vi "Initialize.vi"(7 "laserSettings":T1, 8 "error in (no error)":errorcluster, 10 "dllPath":path, 11 "serialNumber":string) -> (0 "error out":errorcluster, 3 "Laser Diode Controller out":refnum<class "KLD101.lvclass">)   [LabVIEW 2016, in "Laser Diode Controller.lvlib" / "KLD101.lvclass"]
uses:
  KLD101.lvclass
  TypeDefs/KLD-LaserSettings.ctl
  TypeDefs/KLD-LaserMode.ctl
  TypeDefs/KLD-LaserPolarity.ctl
  TypeDefs/KLD-LaserRampMode.ctl
  KLD101.lvclass/KLD101.ctl
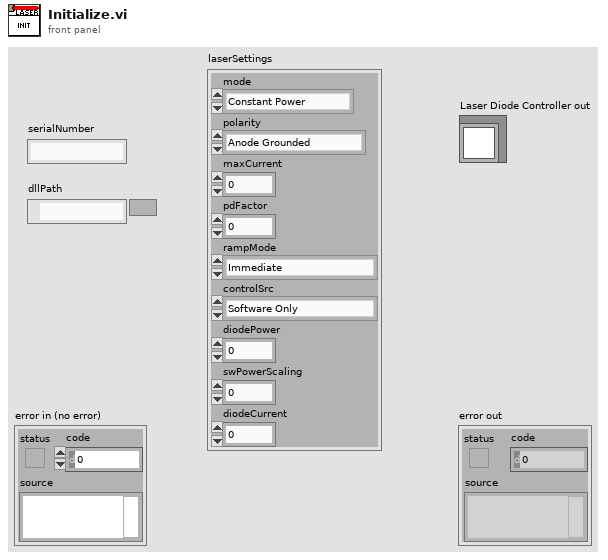
[diagram p1: front panel]
types:
  T1 = typedef "Laser Diode Controller.lvlib/KLD101.lvclass/KLD-LaserSettings.ctl" = cluster{"mode":T2, "polarity":T3, "maxCurrent":i16, "pdFactor":sgl, "rampMode":T4, "controlSrc":enum16{"Software Only", "External Signal", "Potentiometer"}, "diodePower":dbl, "swPowerScaling":dbl, "diodeCurrent":dbl}
  T2 = typedef "Laser Diode Controller.lvlib/KLD101.lvclass/KLD-LaserMode.ctl" = enum16{"Constant Power", "Constant Current"}
  T3 = typedef "Laser Diode Controller.lvlib/KLD101.lvclass/KLD-LaserPolarity.ctl" = enum16{"Anode Grounded", "Cathode Grounded"}
  T4 = typedef "Laser Diode Controller.lvlib/KLD101.lvclass/KLD-LaserRampMode.ctl" = enum16{"Immediate", "Ramped"}
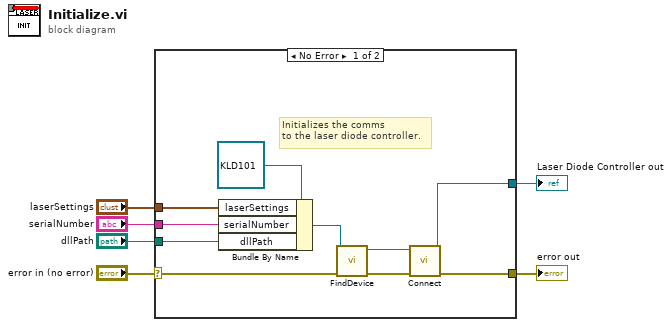
[diagram p0: block diagram]
diagram:
  n1 = case shown="No Error" "error in (no error)" {
    selector: "error in (no error)" -> [w12 w17]
    tunnel: [w8 w17] -> w5
    tunnel: [w10 _] -> w4
    tunnel: "serialNumber" -> [w13 _]
    tunnel: "laserSettings" -> [w15 _]
    tunnel: "dllPath" -> [w7 _]
    frame No Error {
      # "Initializes the comms\nto the laser diode controller."
      n2 = Bundle By Name(cluster=refnum<class "KLD101.lvclass"> refnum ("Laser Diode Controller out"), "laserSettings"=w15, "serialNumber"=w13, "dllPath"=w7) -> (w14:refnum<class "KLD101.lvclass">)
      n3 = call-dynamic "FindDevice.vi"("error in (no error)"=w12, "Laser Diode Controller in"=w14) -> ("error out"=w9:errorcluster, "Laser Diode Controller out"=w11:refnum<class "KLD101.lvclass">)  [unwired: 8 in]
      n4 = call-dynamic "Connect.vi"("error in (no error)"=w9, "Laser Diode Controller in"=w11) -> ("error out"=w8:errorcluster, "Laser Diode Controller out"=w10:refnum<class "KLD101.lvclass">)  [unwired: 8 in]
    }
    frame Error {
    }
  }
  "error out" <- w5
  "Laser Diode Controller out" <- w4
